vi "IndexAndUnbundle.vi"(4 "Index":dbl, 5 "Array":T1(array[cluster]) {"Start" format="%<%.3X>T"}) -> (0 "End":timestamp, 1 "Start":timestamp, 2 "String":string)   [LabVIEW 2017]
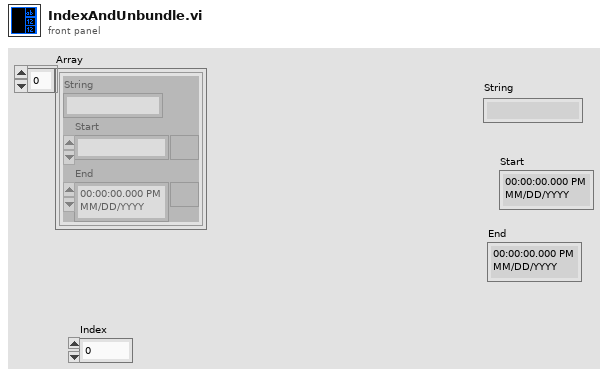
[diagram p1: front panel]
types:
  T1 = cluster{"String":string, "Start":timestamp, "End":timestamp}[]
  T2 = cluster{"String":string, "Start":timestamp, "End":timestamp}
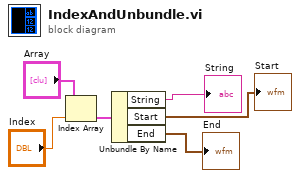
[diagram p0: block diagram]
diagram:
  n1 = Index Array(array="Array", index="Index") -> (element=w4:T2)
  n2 = Unbundle By Name(w4) -> ("String"=→"String":string, "Start"=→"Start":timestamp, "End"=→"End":timestamp)
